vi "Begin.vi"(8 "error in (no error)":errorcluster, 9 "Reverse Solenoid Channel":T1=enum."Solenoid 1", 10 "Forward Solenoid Channel":T1, 11 "DoubleSolenoid in":refnum<class "DoubleSolenoid.lvclass">) -> (0 "error out":errorcluster, 3 "DoubleSolenoid out":refnum<class "DoubleSolenoid.lvclass">)   [LabVIEW 2019, in "Pneumatics control.lvlib" / "DoubleSolenoid.lvclass"]
doc: "This VI opens DoubleSolenoid instance."
uses:
  DoubleSolenoid.lvclass
  C:/Users/rishi/OneDrive/Documents/2020InfinteRecharge/src robot/Classes/Pnematics control/Solenoids/Solenoids.lvclass
  <vilib>/Rock Robotics/WPI/Solenoid/WPI_SolenoidChannel.ctl
  <vilib>/Rock Robotics/WPI/Solenoid/WPI_SolenoidOpenDouble.vi
  Solenoids.lvclass
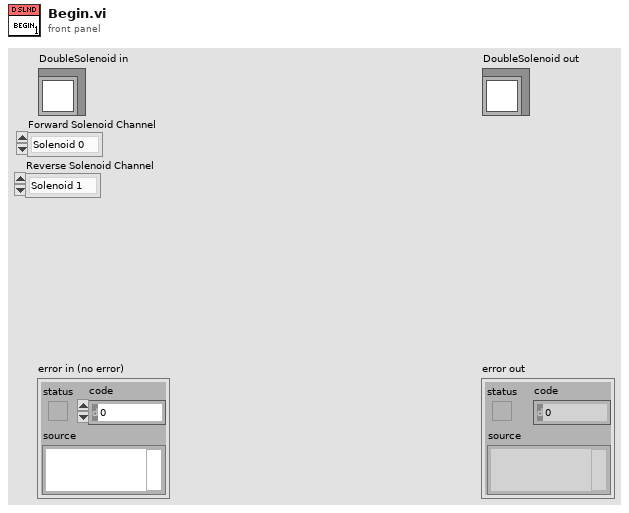
[diagram p1: front panel]
types:
  T1 = typedef "WPI_SolenoidChannel.ctl" = enum8{"Solenoid 0", "Solenoid 1", "Solenoid 2", "Solenoid 3", "Solenoid 4", "Solenoid 5", "Solenoid 6", "Solenoid 7", "Invalid"}
  T2 = typedef "WPI_SolenoidDevRef.ctl" = cluster{"DevStatus":errorcluster, "Pneumatics Control Module":u8, "Forward Solenoid Channel":T1, "Reverse Solenoid Channel":T1}
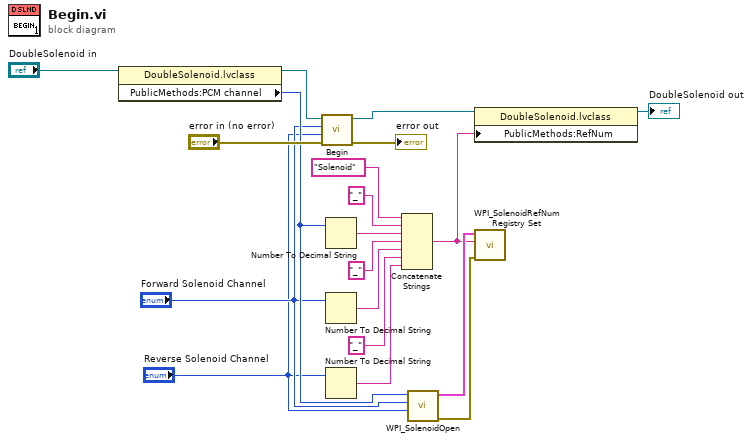
[diagram p0: block diagram]
diagram:
  n1 = property class="DoubleSolenoid.lvclass"(reference="DoubleSolenoid in") -> (reference out=w15:refnum<class "DoubleSolenoid.lvclass">, "PublicMethods:PCM channel"=w14:u8)  [unwired: 1 in, 1 out]
  n2 = call-parent "Begin.vi"("error in (no error)"="error in (no error)", "Reverse solenoid channel"="Reverse Solenoid Channel", "Forward Solenoid Channel"="Forward Solenoid Channel", "Solenoids in"=w15) -> ("error out"=→"error out":errorcluster, "Solenoids out"=w5:refnum<class "DoubleSolenoid.lvclass">)  [unwired: 6 in]
  n3 = Number To Decimal String(number=w14) -> (decimal integer string=w11:string)  [unwired: 1 in]
  n4 = Number To Decimal String(number="Forward Solenoid Channel") -> (decimal integer string=w9:string)  [unwired: 1 in]
  n5 = Number To Decimal String(number="Reverse Solenoid Channel") -> (decimal integer string=w7:string)  [unwired: 1 in]
  n6 = Concatenate Strings("Solenoid" ("string"), "_" ("string"), w11, "_" ("string"), w9, "_" ("string"), w7) -> (w6:string)
  n7 = call-poly <vilib>:"WPI_SolenoidOpen.vi"("Reverse Solenoid Channel"="Reverse Solenoid Channel", "Forward Solenoid Channel"="Forward Solenoid Channel", "Pneumatics Control Module (0)"=w14) -> ("error out"=w16:errorcluster, "SolenoidDevRef"=w17:T2)  [unwired: 7 in]
  n8 = property class="DoubleSolenoid.lvclass"(reference=w5, "PublicMethods:RefNum"=w6) -> (reference out=→"DoubleSolenoid out":refnum<class "DoubleSolenoid.lvclass">)  [unwired: 1 in, 1 out]
  n9 = call <vilib>:"WPI_SolenoidRefNum Registry Set.vi"("error in (no error)"=w16, "refnum name"=w6, "SolenoidDevRef"=w17) -> ()  [unwired: 7 in, 2 out]
